vi "Step 4.vi"(8 "error in (no error)":errorcluster, 11 "HeatUp Data in":string[][](array[string])) -> (0 "error out":errorcluster, 1 "Stabilized Condition":string[][](array[string]), 3 "Max Temp Difference":dbl)   [LabVIEW 2016]
uses:
  <vilib>/Utility/error.llb/DialogType.ctl
panel:
  out "number":dbl
  out "subarray":string[][](array[string])
  out "index of element":i32
  # "Data with Stripped Header"
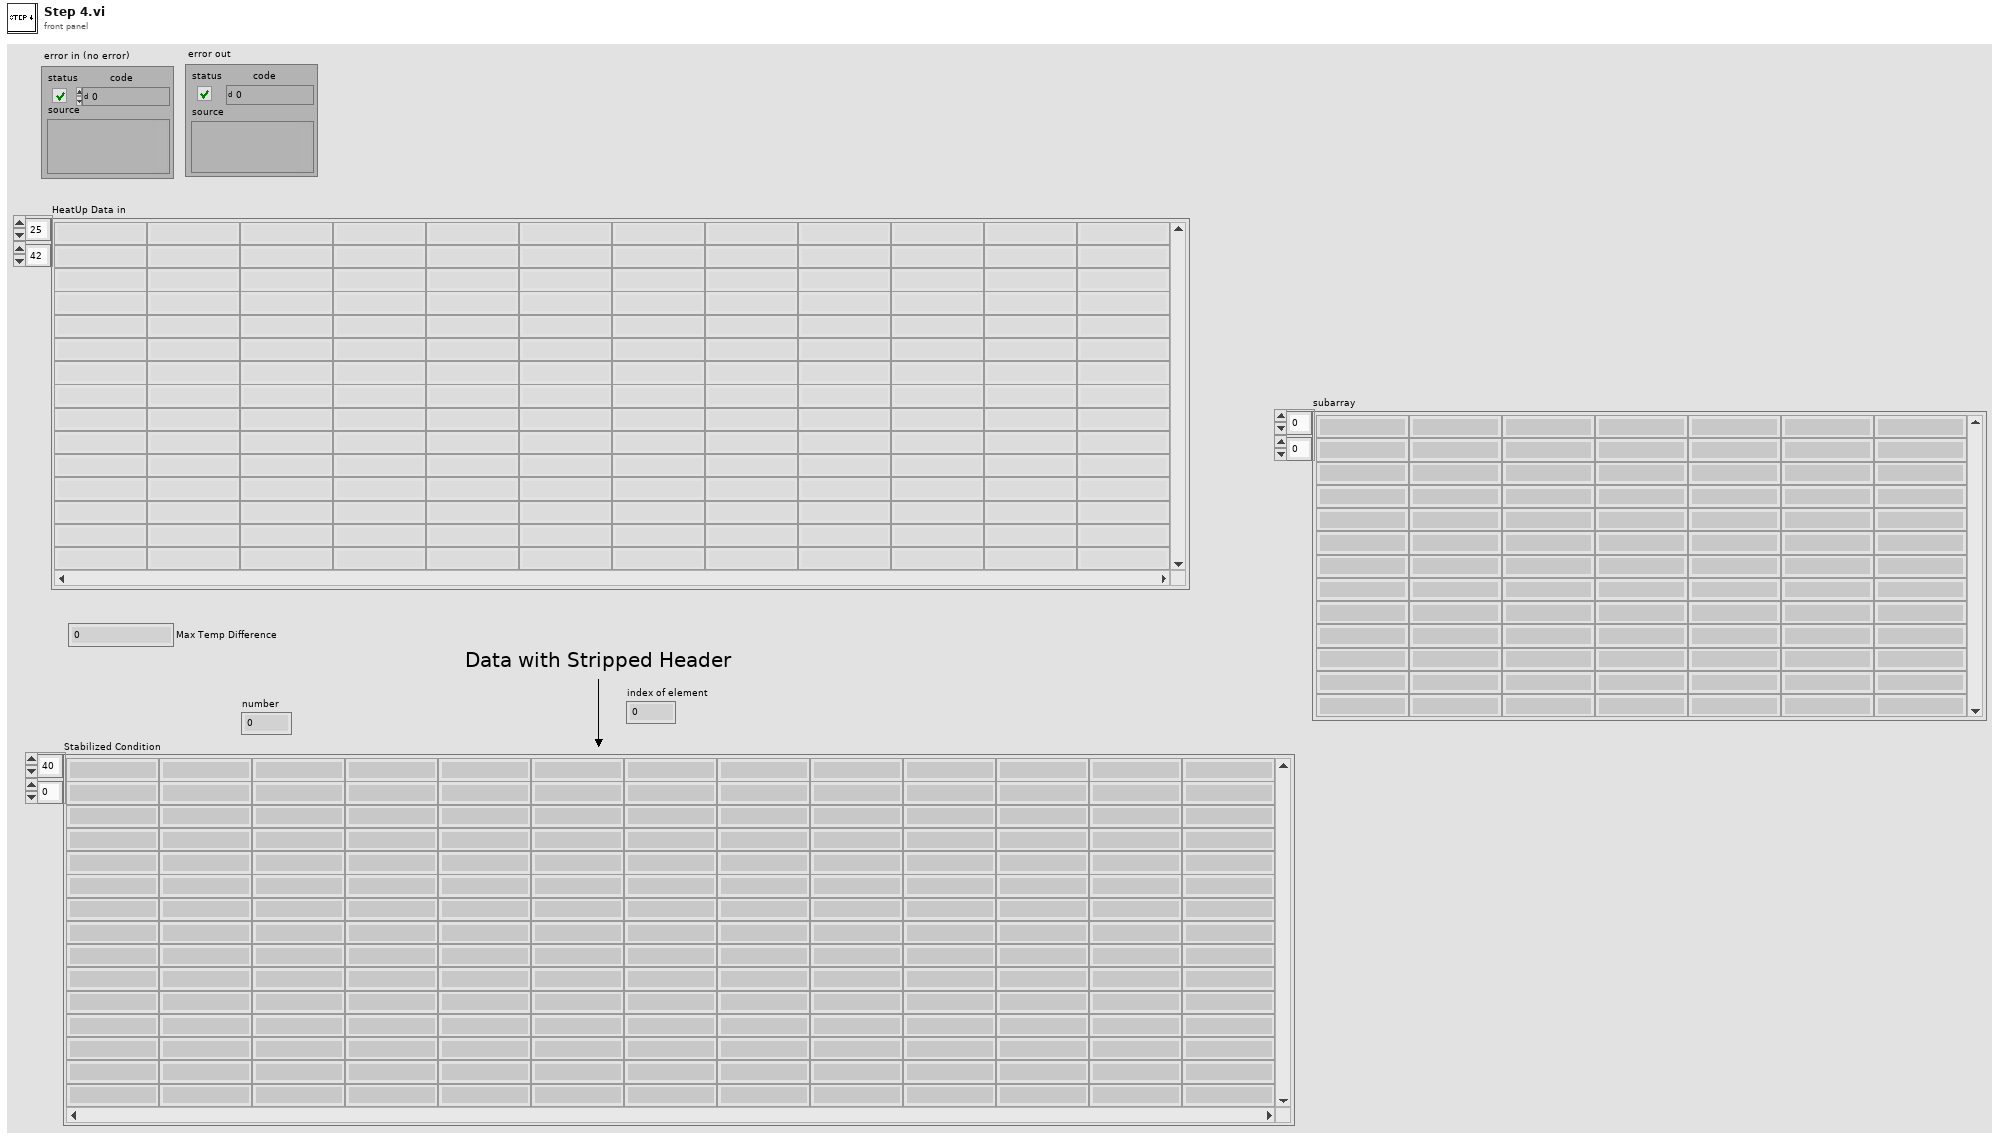
[diagram p1: front panel]
types:
  T1 = typedef "DialogType.ctl" = u16
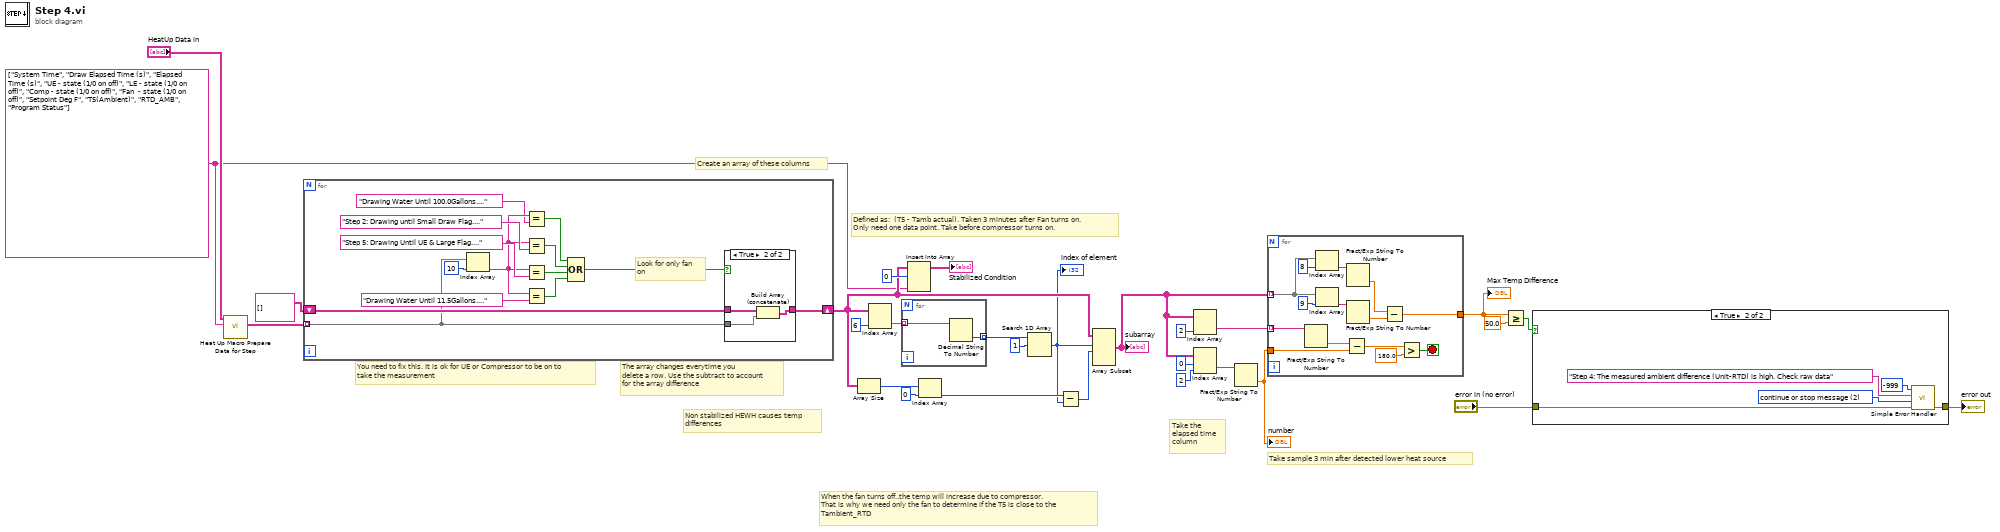
[diagram p0: block diagram]
diagram:
  w1 = string[] ["System Time", "Draw Elapsed Time (s)", "Elapsed Time (s)", "UE - state (1/0 on off)", "LE - state (1/0 on off)", "Comp - state (1/0 on off)", "Fan  - state (1/0 on off)", "Setpoint Deg F", "T5(Ambient)", "RTD_AMB", "Program Status"]
  # "Take sample 3 min after detected lower heat source"
  # "Take the \nelapsed time \ncolumn"
  # "Non stabilized HEWH causes temp\ndifferences"
  # "You need to fix this. It is ok for UE or Compressor to be on to\ntake the measurement"
  # "The array changes everytime you \ndelete a row. Use the subtract to account\nfor the array difference"
  # "When the fan turns off..the temp will increase due to compressor.\nThat is why we need only the fan to determine if the T5 is close to the \nTambient_RTD"
  # "Defined as:  (T5 - Tamb actual). Taken 3 minutes after Fan turns on.\nOnly need one data point. Take before compressor turns on."
  # "Create an array of these columns"
  n1 = call "Heat Up Macro Prepare Data for Step.vi"("Columns Too Search For"=w1, "HeatUp Raw Data Input"="HeatUp Data in") -> ("Heat Up Data with Only Selected Columns"=w2:string[][])  [unwired: 8 in, 1 out]
  n2 = for {
    tunnel: w2 -> [w39] mode=indexing
    shift-right: [w41] -> w17
    shift-left: string[][] [] -> [w42]
    # "Look for only fan\non"
    n3 = Index Array(array=w39, index=10) -> (element=w31:string)
    n4 = Equal?(x=w31, y="Drawing Water Until 100.0Gallons....") -> (x = y?=w29:bool)
    n5 = Equal?(x=w31, y="Step 2: Drawing until Small Draw Flag....") -> (x = y?=w36:bool)
    n6 = Equal?(x=w31, y="Step 5: Drawing Until UE & Large Flag....") -> (x = y?=w37:bool)
    n7 = Equal?(x=w31, y="Drawing Water Until 11.5Gallons....") -> (x = y?=w33:bool)
    n8 = Compound Arithmetic op=OR(w29, w36, w37, w33) -> (w32:bool)
    n9 = case shown="True" w32 {
      tunnel: w42 -> [w43 w46]
      tunnel: [w43 w45] -> w41
      tunnel: w39 -> [_ w44]
      frame False {
      }
      frame True {
        n10 = Build Array (concatenate)(w46, w44) -> (w45:string[][])
      }
    }
  }
  n11 = Array Size(array=w17) -> (size(s)=w16:i32[])
  n12 = Index Array(array=w17, index (col)=6 ("disabled index (col)")) -> (element=w20:string[])  [unwired: 1 in]
  n13 = for {
    tunnel: w20 -> [w48] mode=indexing
    tunnel: [w47] -> w19 mode=indexing
    n14 = Decimal String To Number(string=w48) -> (number=w47:i32)  [unwired: 2 in, 1 out]
  }
  n15 = Insert Into Array(array=w17, index (row)=0, new element=w1) -> (→"Stabilized Condition":string[][])  [unwired: 1 in]
  n16 = Index Array(array=w16, index=0) -> (element=w14:i32)
  n17 = Search 1D Array(1D array=w19, element=1) -> (index of element=w13:i32)  [unwired: 1 in]
  "index of element" <- w13
  n18 = Subtract(x=w14, y=w13) -> (x-y=w12:i32)
  n19 = Array Subset(array=w17, index (row)=w13, length (row)=w12) -> (w5:string[][])  [unwired: 2 in]
  "subarray" <- w5
  n20 = Index Array(array=w5, index (col)=2 ("disabled index (col)")) -> (element=w7:string[])  [unwired: 1 in]
  n21 = Index Array(array=w5, index (row)=0 ("disabled index (row)"), index (col)=2 ("disabled index (col)")) -> (element=w10:string)
  n22 = Fract/Exp String To Number(string=w10) -> (number=w6:dbl)  [unwired: 3 in, 1 out]
  "number" <- w6
  n23 = for {
    tunnel: w7 -> [w62] mode=indexing
    tunnel: w6 -> [w61]
    tunnel: w5 -> [w57] mode=indexing
    tunnel: [w52] -> w4
    stop <- w58 stop-if-true
    n24 = Fract/Exp String To Number(string=w62) -> (number=w49:dbl)  [unwired: 3 in, 1 out]
    n25 = Index Array(array=w57, index=8) -> (element=w54:string)
    n26 = Index Array(array=w57, index=9) -> (element=w53:string)
    n27 = Subtract(x=w49, y=w61) -> (x-y=w60:dbl)
    n28 = Fract/Exp String To Number(string=w54) -> (number=w51:dbl)  [unwired: 3 in, 1 out]
    n29 = Fract/Exp String To Number(string=w53) -> (number=w50:dbl)  [unwired: 3 in, 1 out]
    n30 = Subtract(x=w51, y=w50) -> (x-y=w52:dbl)
    n31 = Greater?(x=w60, y=180.0) -> (0:w58:bool)
  }
  "Max Temp Difference" <- w4
  n32 = Greater Or Equal?(x=w4, y=50.0) -> (x >= y?=w24:bool)
  n33 = case shown="True" w24 {
    tunnel: "error in (no error)" -> [w63 w68]
    tunnel: [w63 w67] -> w26
    frame False {
    }
    frame True {
      w66 = T1 2 items=["no dialog", "OK message", "continue or stop message", "OK message + warnings", "continue/stop + warnings"] ("type of dialog (OK msg:1)")
      n34 = call <vilib>:"Simple Error Handler.vi"("error code (no error:0)"=-999, "error source (\" \")"="Step 4: The measured ambient difference (Unit-RTD) is high. Check raw data" ("error source (\" \")"), "type of dialog (OK msg:1)"=w66, "error in (no error)"=w68) -> ("error out"=w67:errorcluster)  [unwired: 1 in, 4 out]
    }
  }
  "error out" <- w26
